vi "Variant to Limits.vi"(8 "error in":errorcluster, 10 "Setpoint":i32, 11 "Variant":variant) -> (0 "error out":errorcluster, 2 "coerced setpoint":i32)   [LabVIEW 2018, in "IMG_SRC.lvlib" / "IMG_SRC.lvclass"]
uses:
  IMG_SRC.lvclass
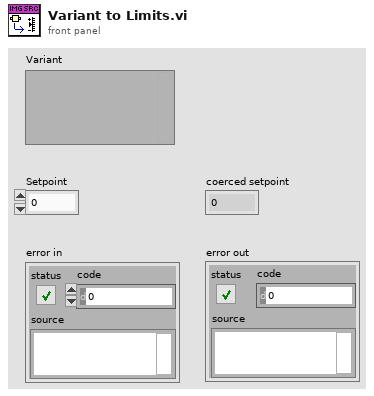
[diagram p1: front panel]
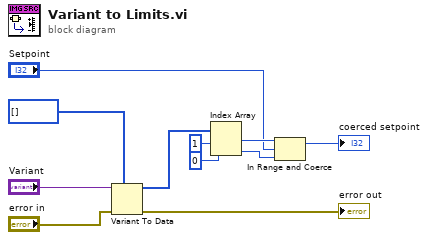
[diagram p0: block diagram]
diagram:
  n1 = Variant To Data(error in="error in", type=i32[] [], Variant="Variant") -> (data=w8:i32[], error out=→"error out":errorcluster)
  n2 = Index Array(array=w8, index #1=1 ("index"), index #2=0 ("index")) -> (element #1=w4:i32, element #2=w3:i32)
  n3 = In Range and Coerce(upper limit=w4, x="Setpoint", lower limit=w3) -> (coerced(x)=→"coerced setpoint":i32)  [unwired: 1 out]
